vi "Create Parent MenuItem.vi"(4 "error in (no error)":errorcluster, 5 "Enabled":bool=TRUE, 6 "Child MenuItems":refnum<k24>[](array[refnum]), 7 "Item Text":string) -> (0 "error out":errorcluster, 3 "MenuItem":refnum<k24>)   [LabVIEW 2020, in "NotifyIcon.lvlib"]
uses:
  NotifyIcon.lvlib
  System.Windows.Forms
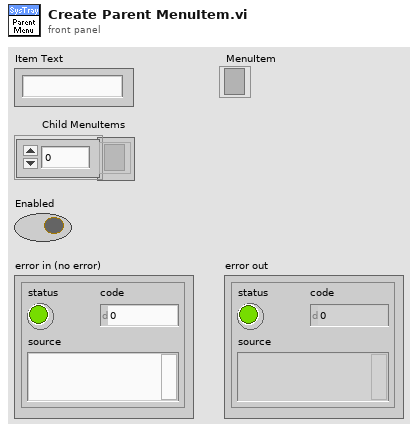
[diagram p1: front panel]
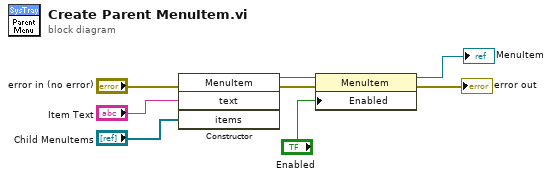
[diagram p0: block diagram]
diagram:
  n1 = constructor class="MenuItem"(error in="error in (no error)", "text"="Item Text", "items"="Child MenuItems") -> (reference out=w2:refnum<k24>, error out=w1:errorcluster)  [unwired: 2 in, 3 out]
  n2 = property class="MenuItem"(reference=w2, error in=w1, "Enabled"="Enabled") -> (reference out=→"MenuItem":refnum<k24>, error out=→"error out":errorcluster)
